vi "Read General CMD.vi"(8 "error in (no error)":errorcluster, 11 "Message in":refnum<class "Message.lvclass">) -> (0 "error out":errorcluster, 2 "General CMD":T1 caption="Enum 3", 3 "Message out":refnum<class "Message.lvclass">)   [LabVIEW 2024, in "Message.lvclass"]
uses:
  Message.lvclass
  Type Def/General CMD.ctl
  Message.lvclass/Message.ctl
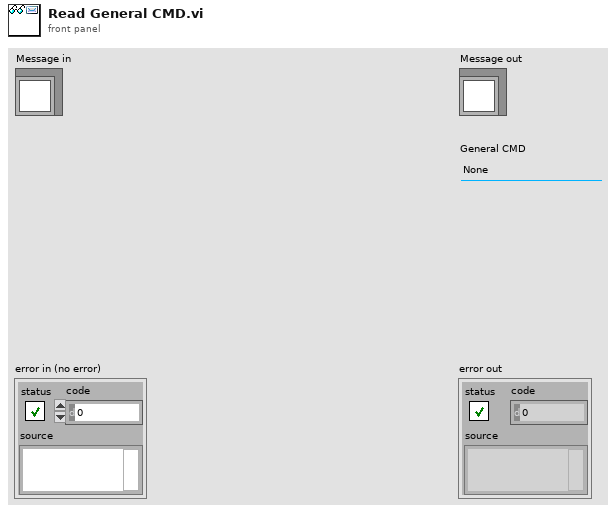
[diagram p1: front panel]
types:
  T1 = typedef "General CMD.ctl" = enum16{"None", "Stop", "Abort", "Running Task", "Running Batch Tasks", "Task Self Running", "Emergency Stop", "Subscribe", "UnSubscribe", "Pause", "Receive Parameters", "Active", "Resume"}
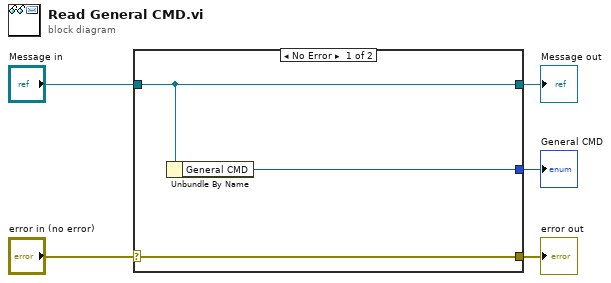
[diagram p0: block diagram]
diagram:
  n1 = case shown="No Error" "error in (no error)" {
    selector: "error in (no error)" -> [w8 w9]
    tunnel: [w8 w9] -> w4
    tunnel: [w7 w10] -> w2
    tunnel: "Message in" -> [w7 w10]
    tunnel: [w6 _] -> w1
    frame No Error {
      n2 = Unbundle By Name(w7) -> ("General CMD"=w6:T1)
    }
    frame Error {
    }
  }
  "error out" <- w4
  "Message out" <- w2
  "General CMD" <- w1
